vi "Real Compact Tri-Matrix Inverse.vi"(0 "Triangular Compact Array":cluster{"Compact Array":dbl[], "array type":i32} {"array type" items=["lower triangular", "upper triangular"]; "Compact Array" format="%.2f"}) -> (1 "Inverse Array":cluster{"Compact Array":dbl[], "array type":i32} {"array type" items=["lower triangular", "upper triangular"]; "Compact Array" format="%.2f"}, 2 "error":i32)   [LabVIEW 2014, in "NI_AALBase.lvlib"]
doc: "Solves a linear system of simultaneous equations, if possible. The system is solved using the method known as L-U decomposition."
uses:
  NI_AALBase.lvlib
  lvanlys.dll
panel:
  # "Real Compact Tri-Matrix Inverse"
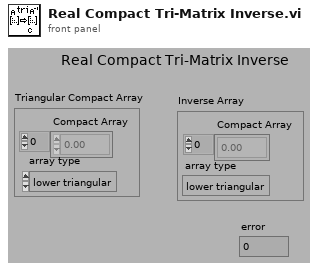
[diagram p1: front panel]
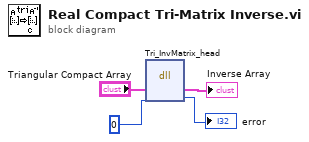
[diagram p0: block diagram]
diagram:
  n1 = dll-call lib="C:/Program Files (x86)/National Instruments/LabVIEW 2014/resource/lvanlys.*" fn="Tri_InvMatrix_head"("Triangular Compact Array"="Triangular Compact Array", 0) -> ("Triangular Compact Array"=→"Inverse Array":cluster{"Compact Array":dbl[], "array type":i32}, →"error":i32)  [unwired: 4 in, 2 out]
